vi "Set Add User.vi"(5 "Access Level":T1(ring), 7 "User Index":i32, 8 "error IO":errorcluster, 9 "Password":string, 10 "User Name":string, 11 "VISA resource name":refnum<visa-resource-name>) -> (0 "error Out":errorcluster, 3 "VISA resource Out":refnum<visa-resource-name>)   [LabVIEW 2012, in "Associated Research 78XX Series.lvlib"]
uses:
  <instrlib>/Associated Research 78XX Series/Associated Research 78XX Series.lvlib
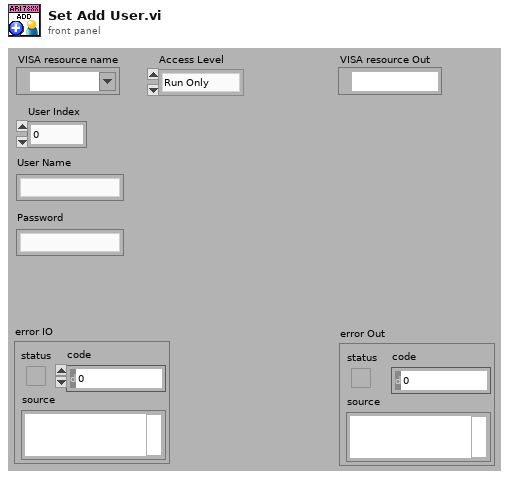
[diagram p1: front panel]
types:
  T1 = enum16{"Run Only", "Recall Setup", "Edit Step", "Full System"}
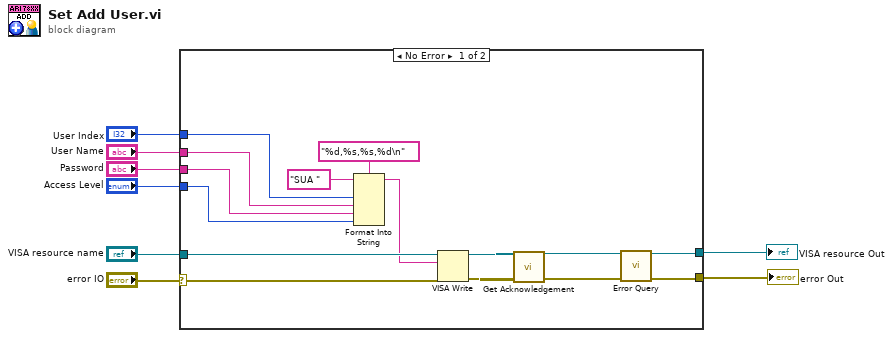
[diagram p0: block diagram]
diagram:
  n1 = case shown="No Error" "error IO" {
    selector: "error IO" -> [w16 w25]
    tunnel: [w22 w25] -> w5
    tunnel: [w23 w24] -> w6
    tunnel: "VISA resource name" -> [w17 w24]
    tunnel: "User Index" -> [w21 _]
    tunnel: "User Name" -> [w20 _]
    tunnel: "Password" -> [w19 _]
    tunnel: "Access Level" -> [w18 _]
    frame No Error {
      n2 = Format Into String(format string="%d,%s,%s,%d\n", initial string="SUA " ("Command to Send (empty)"), w21, w20, w19, w18) -> (resulting string=w11:string)  [unwired: 1 in, 1 out]
      n3 = VISA Write(VISA resource name=w17, write buffer=w11, error in (no error)=w16) -> (VISA resource name out=w9:refnum<visa-resource-name>, error out=w10:errorcluster)  [unwired: 1 out]
      n4 = call <instrlib>:"Get Acknowledgement.vi"("VISA resource name"=w9, "error in (no error)"=w10) -> ("VISA resource name out"=w14:refnum<visa-resource-name>, "error out"=w15:errorcluster)  [unwired: 12 in]
      n5 = call <instrlib>:"Error Query.vi"("VISA resource name"=w14, "error in (no error)"=w15) -> ("VISA resource name out"=w23:refnum<visa-resource-name>, "error out"=w22:errorcluster)  [unwired: 10 in, 2 out]
    }
    frame Error {
    }
  }
  "VISA resource Out" <- w6
  "error Out" <- w5
